vi "Read.vi"(7 "SPI Channel (0)":u8, 8 "Error In (no error)":errorcluster, 9 "Resolution (g)":enum16{"8g", "4g", "2g"}(ring), 10 "CS Channel":u8, 11 "LINX Resource":T1) -> (0 "Error Out":errorcluster, 1 "Temperature":dbl format="%#_3g", 2 "Acceleration Data (g)":T7, 3 "LINX Resource":T1)   [LabVIEW 2020, in "LMH-LINX.lvlib" / "PmodACL2.lvlib"]
doc: "Read acceleration and termperature values from the PmodACL2.\n\nStart by sending a read command 0xB. Next, Send the register you want to read. The first data register is 0xE. Since the first 2 response bytes are empty, we need to send 8 more bytes (2 for each axis and another 2 for temperature) so that we can receive the values.\n\nThe temperature multiplier can vary from person to person. If values are wrong, adjust the multiplier."
uses:
  PmodACL2.lvlib
  Private/Type Defs/LINX Ref.ctl
  Private/Type Defs/Platform.ctl
  Private/Type Defs/Interface.ctl
  Private/Device/Type Defs/LINX Device Config.ctl
  Private/Device/Type Defs/TCP Config.ctl
  Private/Device/Type Defs/Channels.ctl
  Peripherals/SPI/SPI CS Config.ctl
  Private/Type Defs/Peripherals/SPI/SPI CS Logic Level.ctl
  Peripherals/SPI/SPI Write Read 1 Frame.vi
  Peripherals/SPI/SPI Write Read N Frames.vi
  Utilities/Check Channel.vi
  Private/Utilties/Generate Error.vi
  LMH-LINX.lvlib
  Private/Device/Device.lvlib
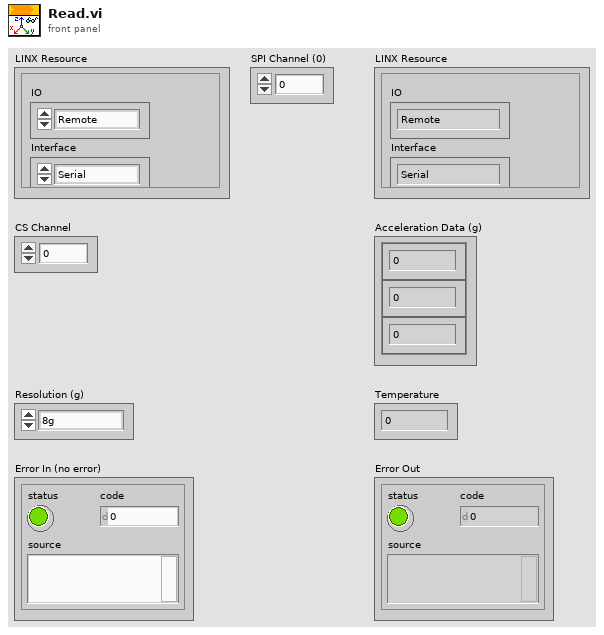
[diagram p1: front panel]
types:
  T1 = typedef "LMH-LINX.lvlib/LINX Ref.ctl" = cluster{"IO":T2, "Interface":T3, "LINX Device Config":T4}
  T2 = typedef "LMH-LINX.lvlib/Platform.ctl" = enum16{"Remote", "Local"}
  T3 = typedef "LMH-LINX.lvlib/Interface.ctl" = enum16{"Serial", "TCP"}
  T4 = typedef "LMH-LINX.lvlib/Device.lvlib/LINX Device Config.ctl" = cluster{"Interface":T3, "COM Port":refnum<visa-resource-name>, "TCP Configuration":T5, "Device Family":u8, "Device ID":u8, "Device Name":string, "TCP Ref":refnum<k5>, "Channels":T6}
  T5 = typedef "LMH-LINX.lvlib/Device.lvlib/TCP Config.ctl" = cluster{"IP Address":string, "Port":u16}
  T6 = typedef "LMH-LINX.lvlib/Channels.ctl" = cluster{"DI":u8[], "DO":u8[], "AI":u8[], "AO":u8[], "PWM":u8[], "QE":u8[], "UART":u8[], "I2C 2":u8[], "SPI":u8[], "CAN":u8[], "Servo":u8[], "AI Ref (V)":dbl, "AI Resolution (Bits)":u8, "AO Ref (V)":dbl, "AO Resolution (Bits)":u8}
  T7 = cluster{"Numeric Control":dbl, "Numeric Control":dbl, "Numeric Control":dbl}
  T8 = typedef "LMH-LINX.lvlib/SPI CS Config.ctl" = cluster{"CS Channel":u8, "CS Logic Level":T9}
  T9 = typedef "LMH-LINX.lvlib/SPI CS Logic Level.ctl" = enum8{"Active Low", "Active High"}
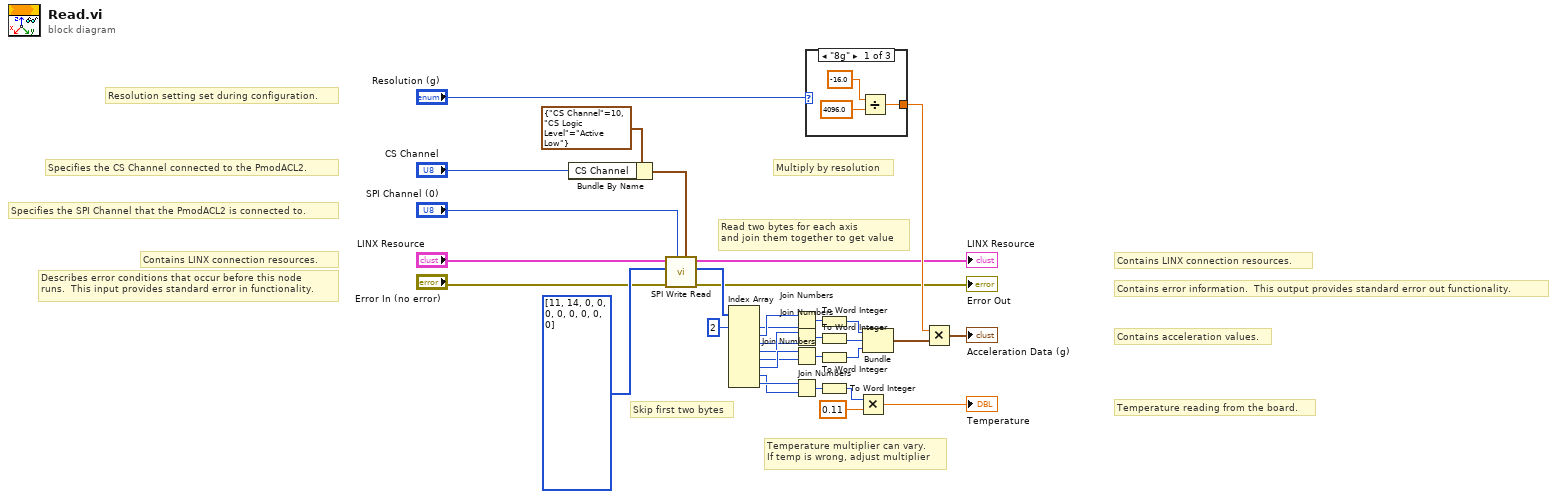
[diagram p0: block diagram]
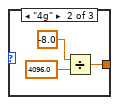
[diagram p2: hidden frame]
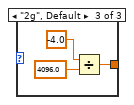
[diagram p3: hidden frame]
diagram:
  # "Temperature multiplier can vary. \nIf temp is wrong, adjust multiplier"
  # "Skip first two bytes"
  # "Read two bytes for each axis\nand join them together to get value"
  # "Multiply by resolution"
  # "Resolution setting set during configuration."
  # "Specifies the CS Channel connected to the PmodACL2."
  # "Temperature reading from the board."
  # "Contains acceleration values."
  # "Contains error information.  This output provides standard error out functionality."
  # "Contains LINX connection resources."
  # "Describes error conditions that occur before this node\nruns.  This input provides standard error in functionality."
  # "Contains LINX connection resources."
  # "Specifies the SPI Channel that the PmodACL2 is connected to."
  n1 = Bundle By Name(cluster=T8 {"CS Channel"=10, "CS Logic Level"=enum."Active Low"} ("CS Configuration"), "CS Channel"="CS Channel") -> (w9:T8)
  n2 = call-poly "SPI Write Read.vi"("CS Configuration"=w9, "SPI Channel (0)"="SPI Channel (0)", "Error In"="Error In (no error)", "Data"=u8[] [11, 14, 0, 0, 0, 0, 0, 0, 0, 0], "LINX Resource"="LINX Resource") -> ("Error Out"=→"Error Out":errorcluster, "Read Data"=w10:u8[], "LINX Resource"=→"LINX Resource":T1)  [unwired: 3 in, 1 out]
  n3 = Index Array(array=w10, index #1=2 ("index")) -> (element #1=w12:u8, element #2=w13:u8, element #3=w15:u8, element #4=w16:u8, element #5=w17:u8, element #6=w18:u8, element #7=w27:u8, element #8=w28:u8)  [unwired: 7 in]
  n4 = Join Numbers(hi=w13, lo=w12) -> ((hi.lo)=w14:u16)
  n5 = Join Numbers(hi=w16, lo=w15) -> ((hi.lo)=w20:u16)
  n6 = Join Numbers(hi=w18, lo=w17) -> ((hi.lo)=w19:u16)
  n7 = Join Numbers(hi=w28, lo=w27) -> ((hi.lo)=w29:u16)
  n8 = case shown="\"8g\"" "Resolution (g)" {
    tunnel: [w34 w37 w40] -> w21
    frame "8g" {
      n9 = Divide(x=-16.0, y=4096.0) -> (x/y=w34:dbl)
    }
    frame "4g" {
      n10 = Divide(x=-8.0, y=4096.0) -> (x/y=w37:dbl)
    }
    frame "2g", Default {
      n11 = Divide(x=-4.0, y=4096.0) -> (x/y=w40:dbl)
    }
  }
  n12 = To Word Integer(number=w14) -> (16bit integer=w22:i16)
  n13 = To Word Integer(number=w20) -> (16bit integer=w23:i16)
  n14 = To Word Integer(number=w19) -> (16bit integer=w24:i16)
  n15 = To Word Integer(number=w29) -> (16bit integer=w30:i16)
  n16 = Multiply(x=w30, y=0.11) -> (x*y=→"Temperature":dbl)
  n17 = Bundle(w22, w23, w24) -> (w25:cluster{i16, i16, i16})  [unwired: 1 in]
  n18 = Multiply(x=w21, y=w25) -> (x*y=→"Acceleration Data (g)":cluster{dbl, dbl, dbl})
